vi "Update Loaded Plugins.vi"(8 "error in (no error)":errorcluster, 10 "Plugin Summary Info":T1[](array[typedef]), 11 "Loaded Plugins ref in":refnum<vi>) -> (0 "error out":errorcluster, 3 "Loaded Plugins ref out":refnum<vi>)   [LabVIEW 2021, in "CIF_UI.lvclass"]
uses:
  CIF_UI.lvclass
  Typedef/Plugin Summary.ctl
  CIFPluginManager/CIFPluginManager/gRPC/CIF_Manager_client/RPC Messages/cif_manager_PluginVersion.ctl
  CIF_UI.lvclass/CIF_UI.ctl
  CIFPluginManager/CIFPluginManager/gRPC/CIF_Manager_client/CIF_Manager_client.lvlib
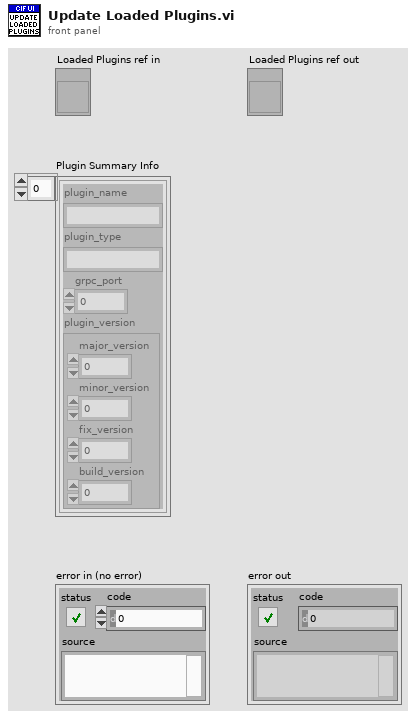
[diagram p1: front panel]
types:
  T1 = typedef "CIF_UI.lvclass/Plugin Summary.ctl" = cluster{"plugin_name":string, "plugin_type":string, "grpc_port":i32, "plugin_version":T2}
  T2 = typedef "CIF_Manager_client.lvlib/cif_manager_PluginVersion.ctl" = cluster{"major_version":i32, "minor_version":i32, "fix_version":i32, "build_version":i32}
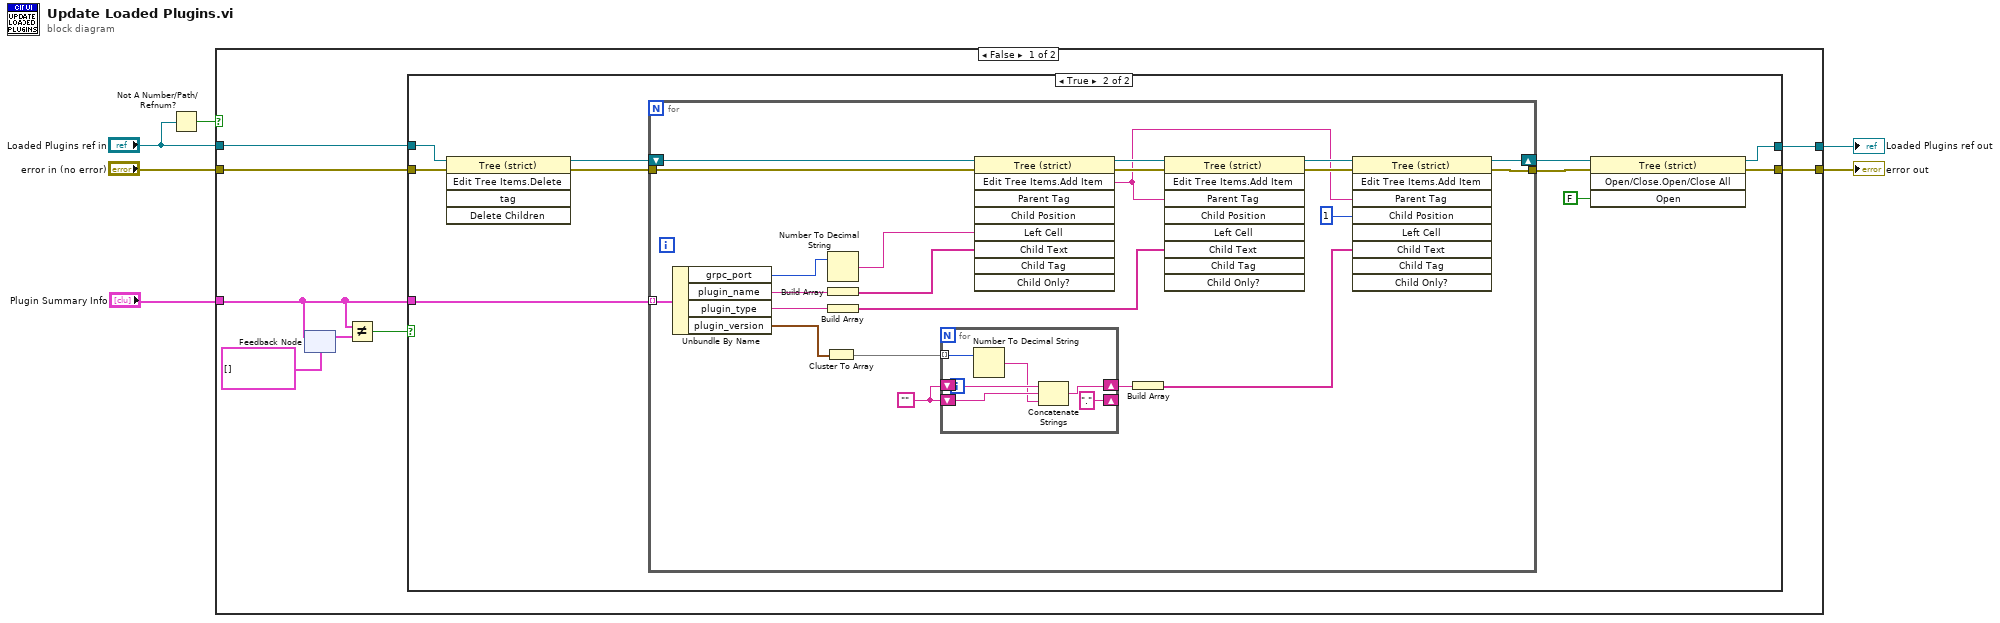
[diagram p0: block diagram]
diagram:
  n1 = Not A Number/Path/Refnum?(number/path/refnum="Loaded Plugins ref in") -> (NaN/Path/Refnum?=w1:bool)
  n2 = case shown="False" w1 {
    tunnel: "error in (no error)" -> [w14 w55]
    tunnel: [w13 w55] -> w5
    tunnel: [w12 w56] -> w4
    tunnel: "Plugin Summary Info" -> [w7 _]
    tunnel: "Loaded Plugins ref in" -> [w11 w56]
    frame False {
      n3 = feedback-in #1(w7) -> ()
      n4 = feedback #1(T1[] [] ("Sorted Plugin Info")) -> (w9:T1[])
      n5 = Not Equal?(x=w7, y=w9) -> (x != y?=w8:bool)
      n6 = case shown="True" w8 {
        tunnel: w14 -> [w15 w21]
        tunnel: [w15 w20] -> w13
        tunnel: [w16 w19] -> w12
        tunnel: w11 -> [w16 w18]
        tunnel: w7 -> [_ w17]
        frame False {
        }
        frame True {
          n7 = invoke class="Tree (strict)" method="Edit Tree Items.Delete"(reference=w18, error in=w21) -> (reference out=w25:refnum<vi>, error out=w26:errorcluster)  [unwired: 3 in, 3 out]
          n8 = for {
            tunnel: w26 -> [w29]
            tunnel: [w48] -> w23
            shift-right: [w45] -> w24
            shift-left: w25 -> [w30]
            tunnel: w17 -> [w31] mode=indexing
            w46 = ""
            n9 = Unbundle By Name(w31) -> ("grpc_port"=w33:i32, "plugin_name"=w32:string, "plugin_type"=w37:string, "plugin_version"=w34:T2)
            n10 = Cluster To Array(cluster=w34) -> (array=w47:i32[])
            n11 = Number To Decimal String(number=w33) -> (decimal integer string=w39:string)  [unwired: 1 in]
            n12 = Build Array(w32) -> (w38:string[])
            n13 = Build Array(w37) -> (w28:string[])
            n14 = for {
              tunnel: w47 -> [w49] mode=indexing
              shift-right: ["."] -> _
              shift-left: w46 -> [w53]
              shift-right: [w51] -> w36
              shift-left: w46 -> [w54]
              n15 = Number To Decimal String(number=w49) -> (decimal integer string=w52:string)  [unwired: 1 in]
              n16 = Concatenate Strings(w54, w53, w52) -> (w51:string)
            }
            n17 = invoke class="Tree (strict)" method="Edit Tree Items.Add Item"(reference=w30, error in=w29, "Left Cell"=w39, "Child Text"=w38) -> (reference out=w44:refnum<vi>, error out=w43:errorcluster, "Edit Tree Items:Add Item"=w27:string)  [unwired: 5 in, 6 out]
            n18 = Build Array(w36) -> (w35:string[])
            n19 = invoke class="Tree (strict)" method="Edit Tree Items.Add Item"(reference=w44, error in=w43, "Parent Tag"=w27, "Child Text"=w28) -> (reference out=w42:refnum<vi>, error out=w41:errorcluster)  [unwired: 5 in, 7 out]
            n20 = invoke class="Tree (strict)" method="Edit Tree Items.Add Item"(reference=w42, error in=w41, "Parent Tag"=w27, "Child Position"=1, "Child Text"=w35) -> (reference out=w45:refnum<vi>, error out=w48:errorcluster)  [unwired: 4 in, 7 out]
          }
          n21 = invoke class="Tree (strict)" method="Open/Close.Open/Close All"(reference=w24, error in=w23, "Open"=FALSE ("Open?")) -> (reference out=w19:refnum<vi>, error out=w20:errorcluster)  [unwired: 1 in, 2 out]
        }
      }
    }
    frame True {
    }
  }
  "Loaded Plugins ref out" <- w4
  "error out" <- w5
